vi "Search for BOM item.vi"(1 "BOM Item":T1, 2 "Inventory":T4[](array[typedef])) -> (0 "Line Item Report":string)   [LabVIEW 2013]
uses:
  Controls/Display Component Line.ctl
  Controls/Components.ctl
  Controls/Component Sub Type.ctl
  Controls/Add Button.ctl
  Controls/Subtract Button.ctl
  BOM Item.ctl
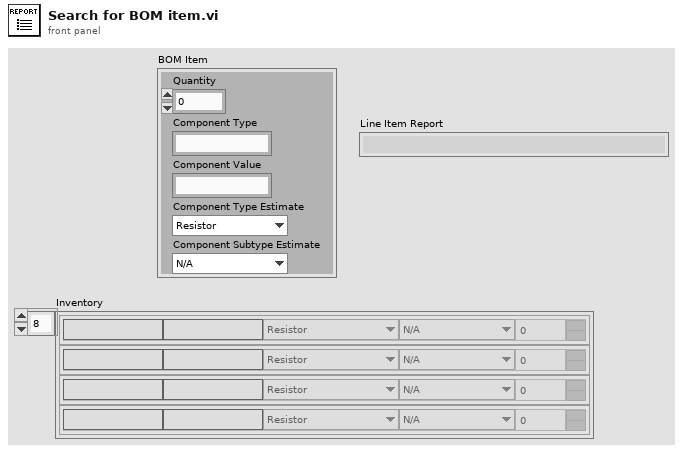
[diagram p1: front panel]
types:
  T1 = typedef "BOM Item.ctl" = cluster{"Quantity":i32, "Component Type":string, "Component Value":string, "Component Type Estimate":T2, "Component Subtype Estimate":T3}
  T2 = typedef "Components.ctl" = enum16{"Resistor", "Capacitor", "Diode", "Voltage Regulator", "Transistors", "ICs", "Misc"}
  T3 = typedef "Component Sub Type.ctl" = enum16{"N/A", "Carbon", "Variable - Trimmer", "Variable - Pot", "Ceramic", "Electrolitic", "Zenner", "TO-92", "TO-220", "NPN", "PNP", "CMOS", "Processor"}
  T4 = typedef "Display Component Line.ctl" = cluster{"Part Number":string, "Code (Value)":string, "Component Type":T2, "Component Subtype":T3, "Quantity":u32, "Add":T5, "Subtract":T6}
  T5 = typedef "Add Button.ctl" = bool
  T6 = typedef "Subtract Button.ctl" = bool
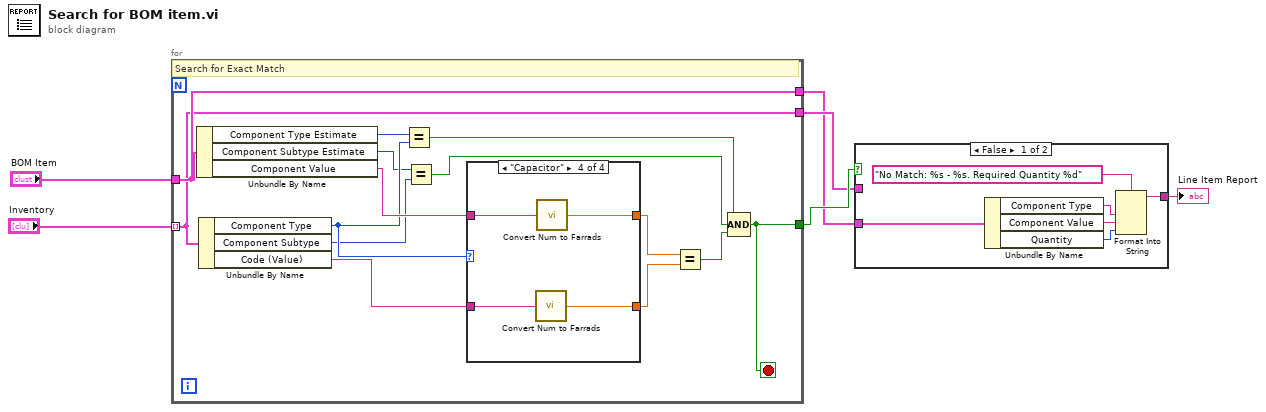
[diagram p0: block diagram]
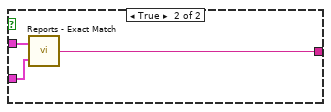
[diagram p2: hidden frame]
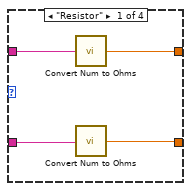
[diagram p3: hidden frame]
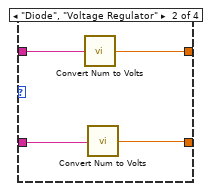
[diagram p4: hidden frame]
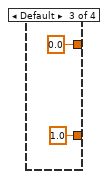
[diagram p5: hidden frame]
diagram:
  n1 = for {
    tunnel: "Inventory" -> [w7] mode=indexing
    tunnel: "BOM Item" -> [w8]
    tunnel: [w9] -> w4
    tunnel: [w8] -> w2
    tunnel: [w7] -> w3
    stop <- w9 stop-if-true
    # "Search for Exact Match"
    n2 = Unbundle By Name(w8) -> ("Component Type Estimate"=w18:T2, "Component Subtype Estimate"=w16:T3, "Component Value"=w20:string)
    n3 = Unbundle By Name(w7) -> ("Component Type"=w17:T2, "Component Subtype"=w15:T3, "Code (Value)"=w19:string)
    n4 = Equal?(x=w18, y=w17) -> (x = y?=w10:bool)
    n5 = Equal?(x=w16, y=w15) -> (x = y?=w11:bool)
    n6 = case shown="\"Capacitor\"" w17 {
      tunnel: w20 -> [w24 w27 _ w34]
      tunnel: w19 -> [w23 w28 _ w33]
      tunnel: [w21 w26 0.0 ("Numeric") w32] -> w14
      tunnel: [w22 w25 1.0 ("Numeric") w31] -> w13
      frame "Resistor" {
        n7 = call "Convert Num to Ohms.vi"("String"=w24) -> ("Numeric"=w21:dbl)
        n8 = call "Convert Num to Ohms.vi"("String"=w23) -> ("Numeric"=w22:dbl)
      }
      frame "Diode", "Voltage Regulator" {
        n9 = call "Convert Num to Volts.vi"("String"=w27) -> ("Numeric"=w26:dbl)
        n10 = call "Convert Num to Volts.vi"("String"=w28) -> ("Numeric"=w25:dbl)
      }
      frame Default {
      }
      frame "Capacitor" {
        n11 = call "Convert Num to Farrads.vi"("String"=w33) -> ("Numeric"=w31:dbl)
        n12 = call "Convert Num to Farrads.vi"("String"=w34) -> ("Numeric"=w32:dbl)
      }
    }
    n13 = Equal?(x=w14, y=w13) -> (x = y?=w12:bool)
    n14 = Compound Arithmetic op=AND(w10, w11, w12) -> (w9:bool)
  }
  n15 = case shown="False" w4 {
    tunnel: w3 -> [_ w42]
    tunnel: w2 -> [w40 w43]
    tunnel: [w35 w41] -> w1
    frame False {
      n16 = Unbundle By Name(w40) -> ("Component Type"=w38:string, "Component Value"=w37:string, "Quantity"=w36:i32)
      n17 = Format Into String(format string="No Match: %s - %s. Required Quantity %d", w38, w37, w36) -> (resulting string=w35:string)  [unwired: 2 in, 1 out]
    }
    frame True {
      n18 = call "Reports - Exact Match.vi"("BOM Item"=w43, "Inventory Item"=w42) -> ("Line Item Report"=w41:string)
    }
  }
  "Line Item Report" <- w1
